vi "Filter_String_Parser.vi"(8 "error in":errorcluster, 11 "Filter String":string="Protocol == UDP AND Length > 0.7 OR Source == 192.168.1.1") -> (0 "error constant":errorcluster, 1 "Comparators":T1(array[cluster]), 3 "Boolean Connectors":string[](array[string]))   [LabVIEW 2025, in "Automotive Ethernet Bus Monitor UI.lvlib" / "Table_Filtering.lvlib"]
uses:
  Table_Filtering.lvlib
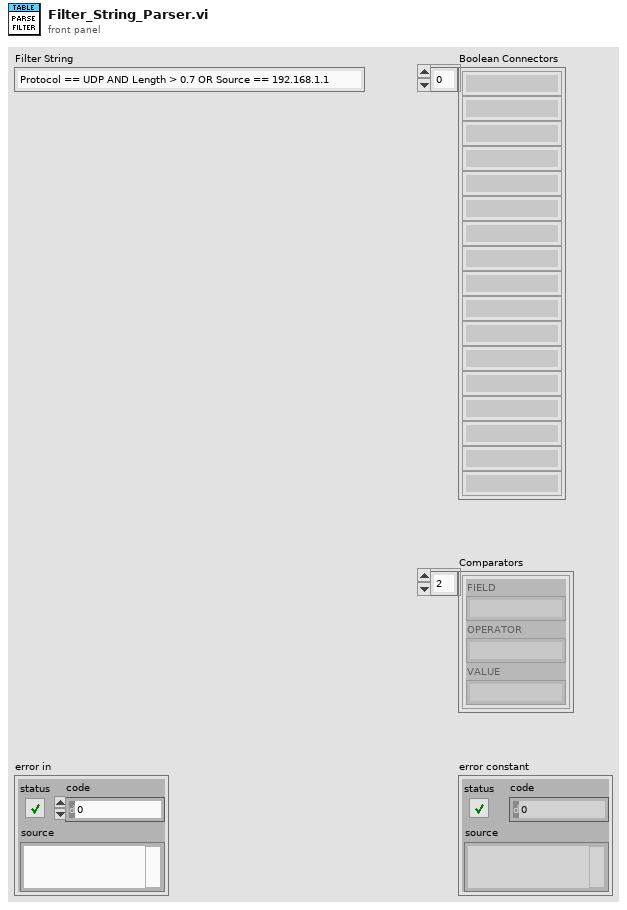
[diagram p1: front panel]
types:
  T1 = cluster{"FIELD":string, "OPERATOR":string, "VALUE":string}[]
  T2 = enum16{"Packet Number", "Timestamp", "Source", "Destination", "Protocol", "Length", "Data"}
  T3 = cluster{"FIELD":string, "OPERATOR":string, "VALUE":string}
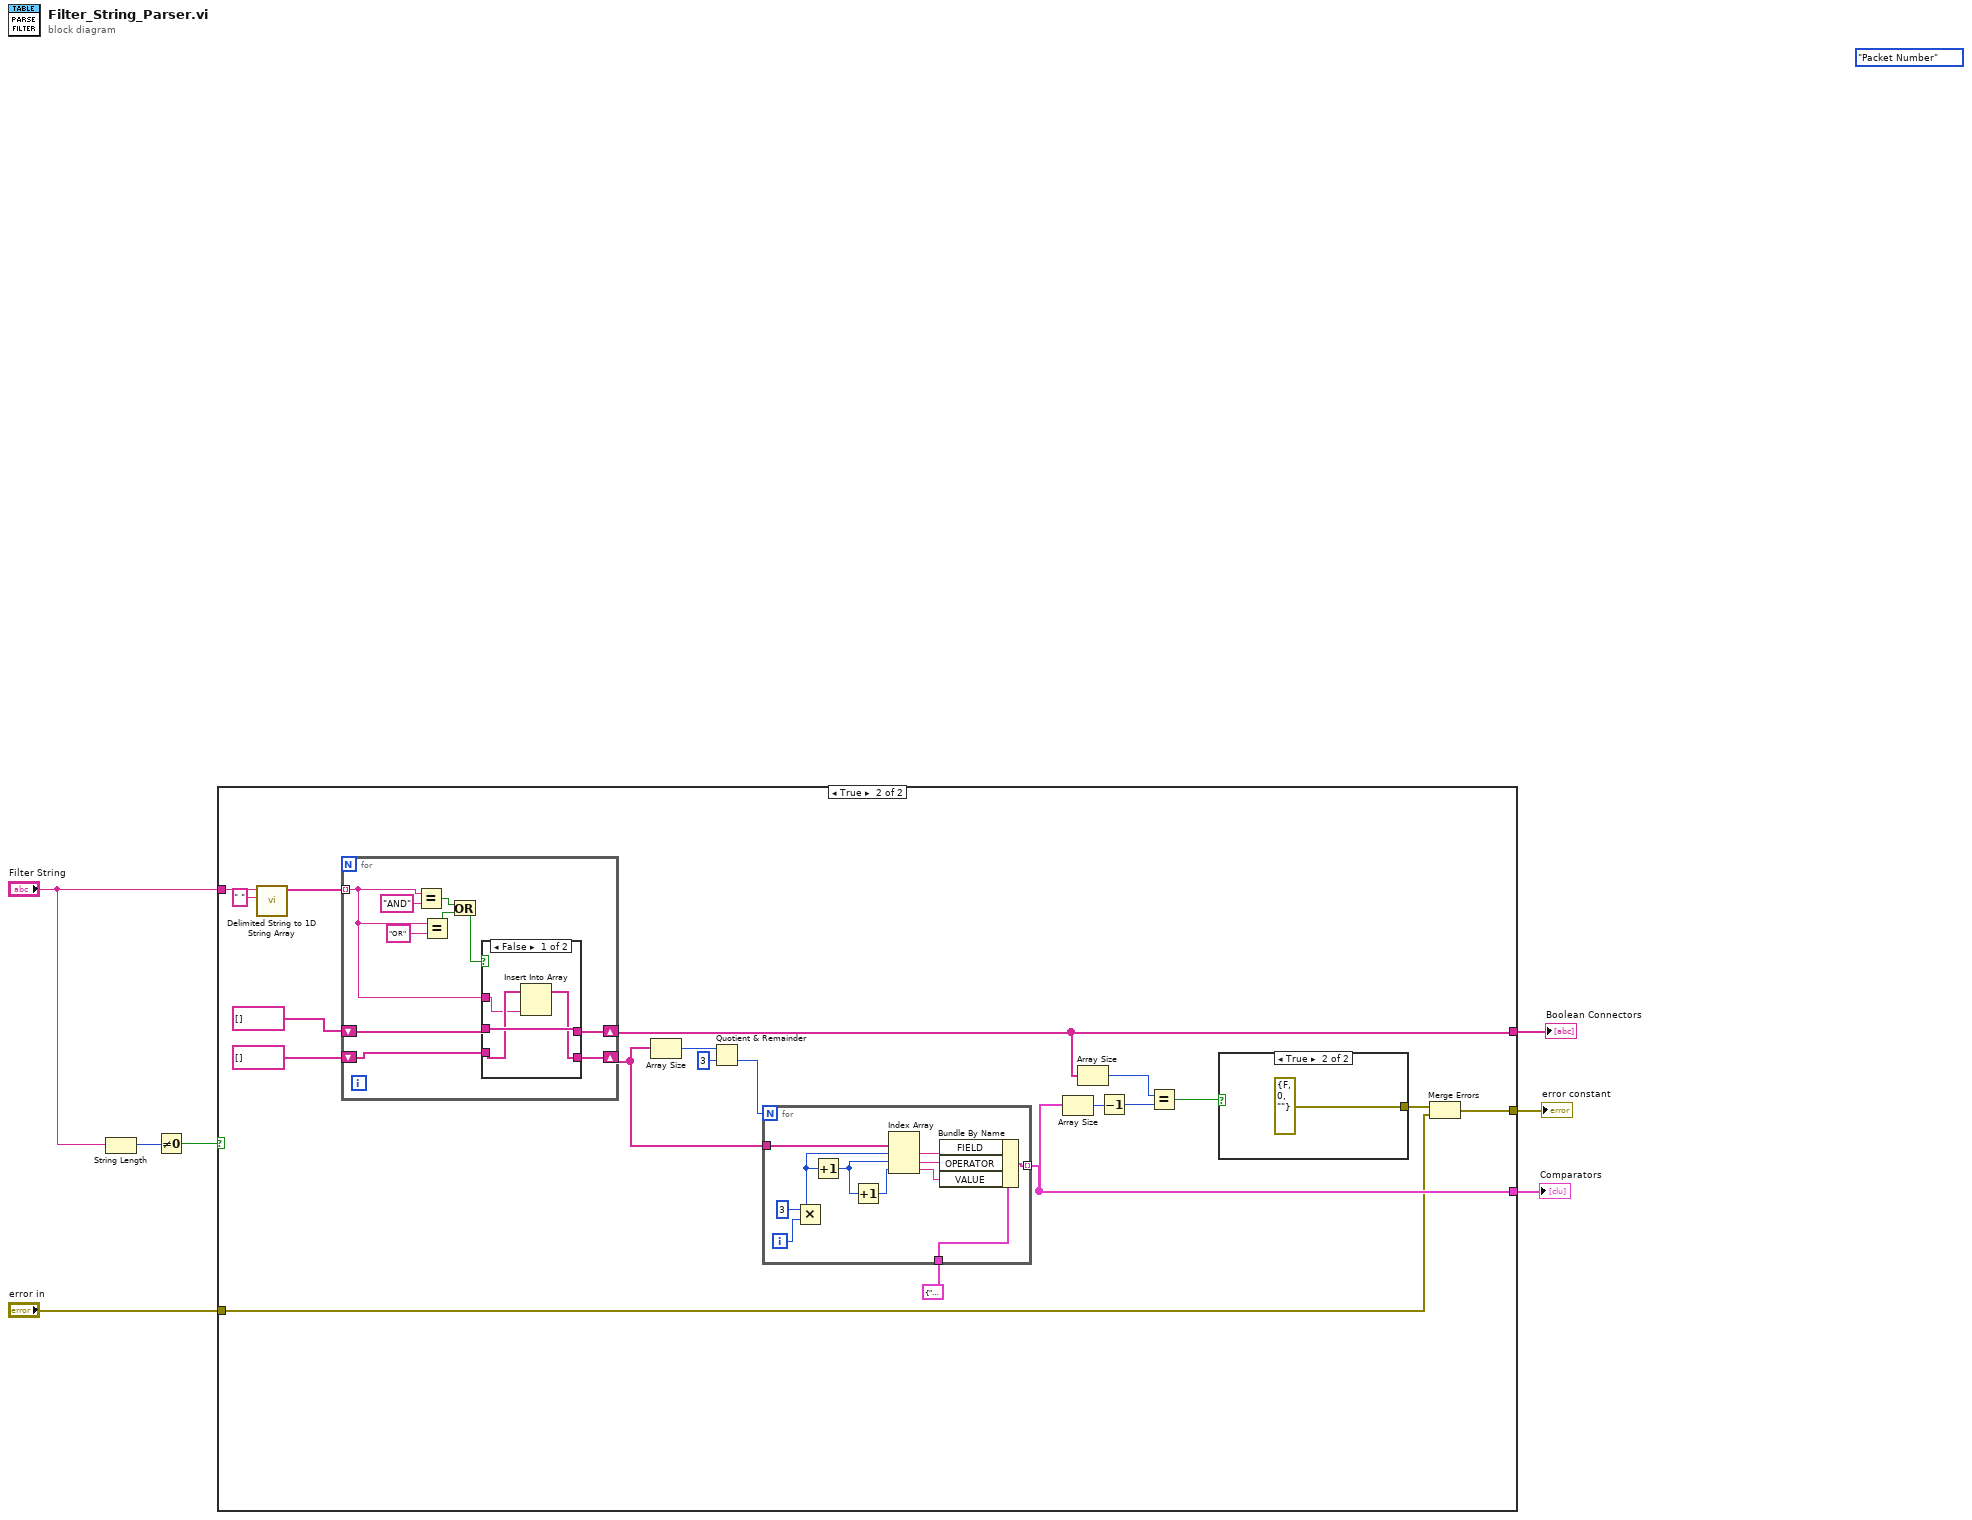
[diagram p0: block diagram]
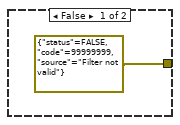
[diagram p3: hidden frame]
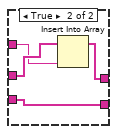
[diagram p4: hidden frame]
diagram:
  (unwired) T2."Packet Number" ("Sort By")
  n1 = String Length(string="Filter String") -> (length=w6:i32)
  n2 = Not Equal To 0?(x=w6) -> (x != 0?=w5:bool)
  n3 = case shown="True" w5 {
    tunnel: "Filter String" -> [_ w18]
    tunnel: [_ w17] -> w4
    tunnel: [_ w14] -> w3
    tunnel: [w8 w11] -> w2
    tunnel: "error in" -> [w8 w9]
    frame False {
    }
    frame True {
      n4 = call <vilib>:"Delimited String to 1D String Array.vi"("delimiter"=" ", "delimited string"=w18) -> ("string array"=w26:string[])  [unwired: 9 in]
      n5 = for {
        tunnel: w26 -> [w45] mode=indexing
        shift-right: [w41] -> w14
        shift-left: string[] [] -> [w44]
        shift-right: [w42] -> w21
        shift-left: string[] [] -> [w43]
        n6 = Equal?(x=w45, y="AND") -> (x = y?=w50:bool)
        n7 = Equal?(x=w45, y="OR") -> (x = y?=w47:bool)
        n8 = Or(x=w50, y=w47) -> (x .or. y?=w46:bool)
        n9 = case shown="False" w46 {
          tunnel: w45 -> [w52 w56]
          tunnel: w44 -> [w54 w57]
          tunnel: [w54 w55] -> w41
          tunnel: w43 -> [w53 w58]
          tunnel: [w51 w58] -> w42
          frame False {
            n10 = Insert Into Array(array=w53, new element=w52) -> (w51:string[])  [unwired: 1 in]
          }
          frame True {
            n11 = Insert Into Array(array=w57, new element=w56) -> (w55:string[])  [unwired: 1 in]
          }
        }
      }
      n12 = Array Size(array=w21) -> (size(s)=w24:i32)
      n13 = Quotient & Remainder(x=w24, y=3) -> (floor(x/y)=w19:i32)  [unwired: 1 out]
      n14 = for {
        N: w19 -> [_]
        tunnel: w21 -> [w40]
        tunnel: T3 {"FIELD"="", "OPERATOR"="", "VALUE"=""} -> [w34]
        tunnel: [w30] -> w17 mode=indexing
        i -> [w39]
        n15 = Multiply(x=3, y=w39) -> (x*y=w37:i32)
        n16 = Increment(x=w37) -> (x+1=w35:i32)
        n17 = Increment(x=w35) -> (x+1=w36:i32)
        n18 = Index Array(array=w40, index #1=w37, index #2=w35, index #3=w36) -> (element #1=w33:string, element #2=w32:string, element #3=w31:string)
        n19 = Bundle By Name(cluster=w34, "FIELD"=w33, "OPERATOR"=w32, "VALUE"=w31) -> (w30:T3)
      }
      n20 = Array Size(array=w17) -> (size(s)=w15:i32)
      n21 = Array Size(array=w14) -> (size(s)=w16:i32)
      n22 = Decrement(x=w15) -> (x-1=w13:i32)
      n23 = Equal?(x=w16, y=w13) -> (x = y?=w12:bool)
      n24 = case shown="True" w12 {
        tunnel: [errorcluster {"status"=FALSE, "code"=99999999, "source"="Filter not valid"} ("error constant") errorcluster {"status"=FALSE, "code"=0, "source"=""} ("error constant")] -> w10
        frame False {
        }
        frame True {
        }
      }
      n25 = Merge Errors(w10, w9) -> (w11:errorcluster)
    }
  }
  "Boolean Connectors" <- w3
  "Comparators" <- w4
  "error constant" <- w2
